vi "GetImage.vi"() -> ()   [LabVIEW 2014]
uses:
  <vilib>/Utility/sysdir.llb/System Directory Type.ctl
  <vilib>/FTP/NI_FTP.lvlib
panel:
  out "data":string
  out "Image":T1(plugin-control)
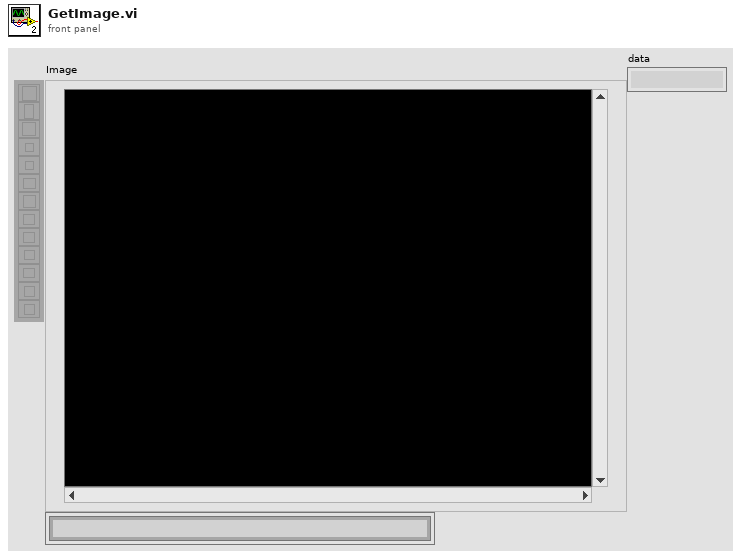
[diagram p1: front panel]
types:
  T1 = typedef "IMAQ Image.ctl" = refnum<image>
  T2 = typedef "System Directory Type.ctl" = i32
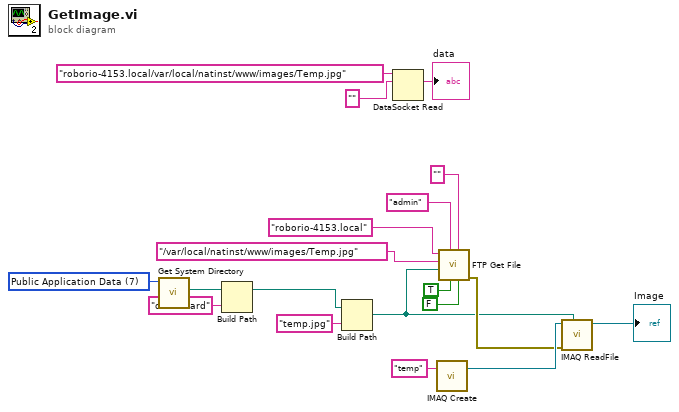
[diagram p0: block diagram]
diagram:
  w17 = T2 7 items=["User Home"=0, "User Desktop"=1, "User Documents"=2, "User Application Data"=3, "User Preferences"=4, "User Temporary"=5, "Public Documents"=6, "Public Application Data"=7, "Public Preferences"=8, "Public Cache"=13, "System Core Libraries"=9, "System Installed Libraries"=10, "Application Files"=11, "Boot Volume Root"=12] ("system directory type")
  n1 = call <vilib>:"Get System Directory.vi"("system directory type"=w17) -> ("system directory"=w16:path)  [unwired: 10 in]
  n2 = Build Path(base path=w16, name or relative path="dashboard") -> (appended path=w5:path)
  n3 = Build Path(base path=w5, name or relative path="temp.jpg") -> (appended path=w11:path)
  n4 = DataSocket Read(10:"" ("password"), 11:"roborio-4153.local/var/local/natinst/www/images/Temp.jpg" ("connection in")) -> (2:→"data":string)  [unwired: 3 in, 6 out]
  n5 = call "IMAQ Create"("Image Name"="temp") -> ("New Image"=w13:T1)  [unwired: 4 in, 1 out]
  n6 = call <vilib>:"FTP Get File.vi"("active (T)"=FALSE, "password"="", "binary (F)"=TRUE, "user"="admin", "local path"=w11, "remote path"="/var/local/natinst/www/images/Temp.jpg", "host"="roborio-4153.local") -> ("error out"=w12:errorcluster)  [unwired: 3 in, 1 out]
  n7 = call "IMAQ ReadFile"("File Path"=w11, "error in (no error)"=w12, "Image"=w13) -> ("Image Out"=→"Image":T1)  [unwired: 4 in, 4 out]
